vi "Funct acq pre-checks.vi"() -> (1 "Proceed":bool)   [LabVIEW 2013]
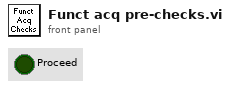
[diagram p1: front panel]
types:
  T1 = typedef "Fixed strings.ctl" = cluster{"ROI file name":string, "Normalised ROI file name":string, "Zplane Pockels values file name":string, "Functional data folder name":string, "Experiment Header file name":string, "Z-stack images folder name":string, "Groups setup rel. path":string, "Groups text file rel. path":string, "TDMS files folder name (F.img)":string, "TDMS files folder name (V.acq)":string, "TDMS files folder name (Pl.acq)":string, "Cycle rel times sequence file":string, "Dynamically called VIs folder name":string, "Time Series folder base name":string}
  T2 = typedef "AOL_Globals.ctl" = cluster{"Imaging Protocol":T3, "Number of POI":u16, "Number of Miniscans":u16, "Number of Trials":u16, "Number of Cycles ":u64, "# Averaged Frames":u16, "Laser power (%)":u8, "Pockels":dbl, "Acquisition Length (sec)":dbl, "Fill time (us)":dbl, "POI Dwell time (us)":dbl, "Miniscan Dwell time per pixel (us)":dbl, "PMT 1":dbl, "PMT 2":dbl, "Back Apperture":dbl, "Frame Size":T4, "Center Frequency":dbl, "Field of View":dbl, "DwellTime (us)":dbl, "Wavelength (nm)":dbl, "Zoom":dbl, "AOL Z":dbl, "AOL Mode":T5, "GridXY":dbl, "GridZ":dbl, "TriggerPeriod (sec)":dbl, "Number of Pixels in Miniscan":u16, "Experiment folder path":path, "X centre":dbl, "Y centre":dbl, "Angle (degrees)":dbl, "Plane Mode":T6, "Threshold":u16[], "Regenerate Chirps":bool, "Rectangle ROI length (pixels)":u16, "Rectangle ROI height (pixels)":u16, "AOD fill":u16, "Samples Wait after Trigger":u16, "StartUp Delay":i32, "Slip Cycle":u32, "Add Cycle":bool}
  T3 = typedef "Imaging Protocols enum.ctl" = enum16{"AOL Z-Stack", "Motor Z Stack", "Functional Acquisition", "Single Plane Acquisition", "Volume Acquisition", "Live Imaging", "Live Plane Imaging", "Live Volume Imaging"}
  T4 = typedef "Frame Size.ctl" = u16
  T5 = typedef "AOL modes.ctl" = enum16{"Raster", "Structural", "Pointing", "Mini Scan", "Alignment"}
  T6 = typedef "Plane Mode.ctl" = u16
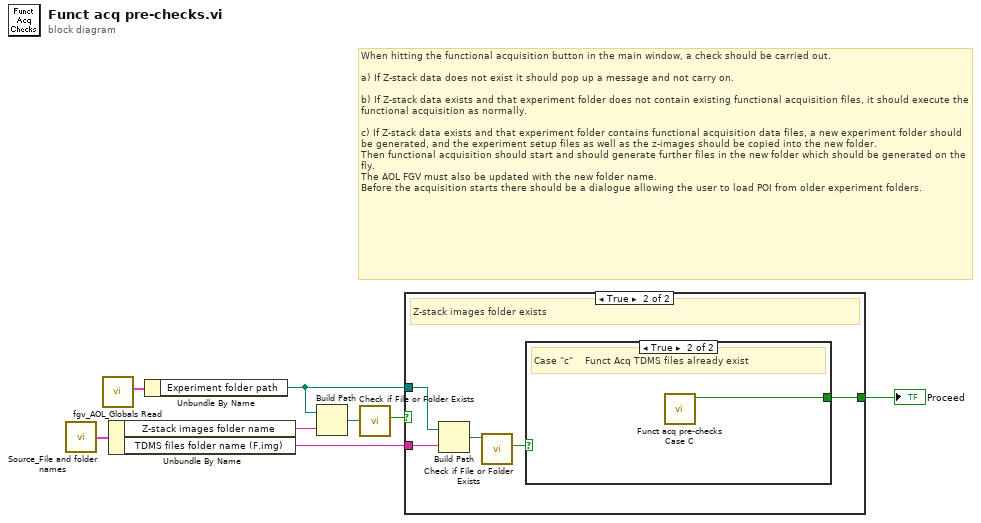
[diagram p0: block diagram]
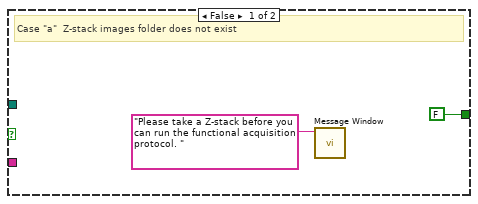
[diagram p2: hidden frame]
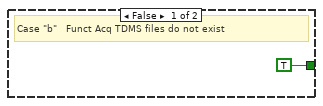
[diagram p3: hidden frame]
diagram:
  # "When hitting the functional acquisition button in the main window, a check should be carried out.\n\na) If Z-stack data does not exist it should pop up a message and not carry on.\n\nb) If Z-stack data exists and that experiment folder does not contain existing functional acquisition files, it should execute the functional acquisition as normally.\n\nc) If Z-stack data exists and that experiment folder contains functional acquisition data files, a new experiment folder should be generated, and the experiment setup files as well as the z-images should be copied into the new folder. \nThen functional acquisition should start and should generate further files in the new folder which should be generated on the fly. \nThe AOL FGV must also be updated with the new folder name. \nBefore the acquisition starts there should be a dialogue allowing the user to load POI from older experiment folders."
  n1 = call "Source_File and folder names.vi"() -> ("Fixed strings"=w7:T1)  [unwired: 1 in]
  n2 = call "fgv_AOL_Globals Read.vi"() -> ("AOL_Globals"=w8:T2)  [unwired: 9 in, 2 out]
  n3 = Unbundle By Name(w7) -> ("Z-stack images folder name"=w6:string, "TDMS files folder name (F.img)"=w1:string)
  n4 = Unbundle By Name(w8) -> ("Experiment folder path"=w2:path)
  n5 = Build Path(base path=w2, name or relative path=w6) -> (appended path=w5:path)
  n6 = call <vilib>:"Check if File or Folder Exists.vi"("path"=w5) -> ("file or folder exists?"=w4:bool)  [unwired: 8 in, 2 out]
  n7 = case shown="True" w4 {
    tunnel: [FALSE w11] -> w3
    tunnel: w2 -> [_ w15]
    tunnel: w1 -> [_ w14]
    frame False {
      # "Case \"a\"  Z-stack images folder does not exist"
      n8 = call "Message Window.vi"("Message string"="Please take a Z-stack before you can run the functional acquisition protocol. ") -> ()  [unwired: 10 in, 1 out]
    }
    frame True {
      # "Z-stack images folder exists"
      n9 = Build Path(base path=w15, name or relative path=w14) -> (appended path=w13:path)
      n10 = call <vilib>:"Check if File or Folder Exists.vi"("path"=w13) -> ("file or folder exists?"=w12:bool)  [unwired: 8 in, 2 out]
      n11 = case shown="True" w12 {
        tunnel: [TRUE w17] -> w11
        frame False {
          # "Case \"b\"   Funct Acq TDMS files do not exist"
        }
        frame True {
          # "Case \"c\"    Funct Acq TDMS files already exist"
          n12 = call "Funct acq pre-checks Case C.vi"() -> ("Proceed"=w17:bool)  [unwired: 11 in]
        }
      }
    }
  }
  "Proceed" <- w3
